vi "Parse JSON for Channels.vi"(7 "Settings(JSON)":string, 8 "error in":errorcluster) -> (0 "error out":errorcluster, 1 "Channel Paths":string[](array[string]), 2 "Channel TypeNames":string[](array[string]), 3 "Channel JSONs":string[](array[string]), 5 "Settings(JSON)":string)   [LabVIEW 2026, in "NIDMM Deployment Hooks.lvlib"]
uses:
  NIDMM Deployment Hooks.lvlib
  <vilib>/JDP Science/JSONtext/JSONtext.lvlib
  <vilib>/regexp/Match Regular Expression.xnode
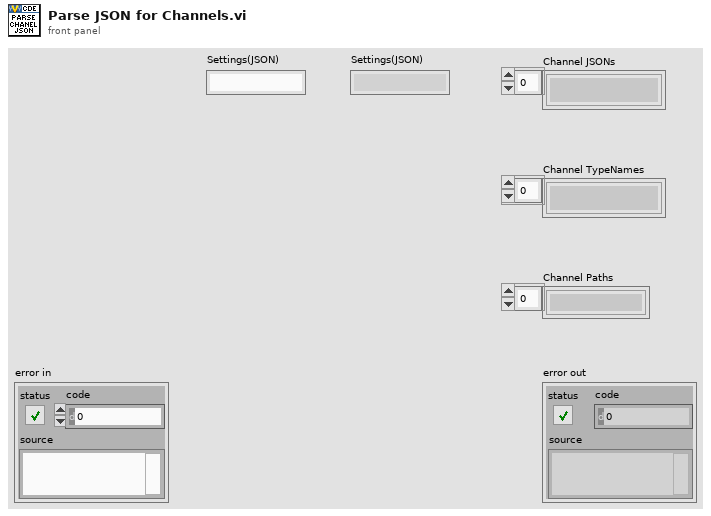
[diagram p1: front panel]
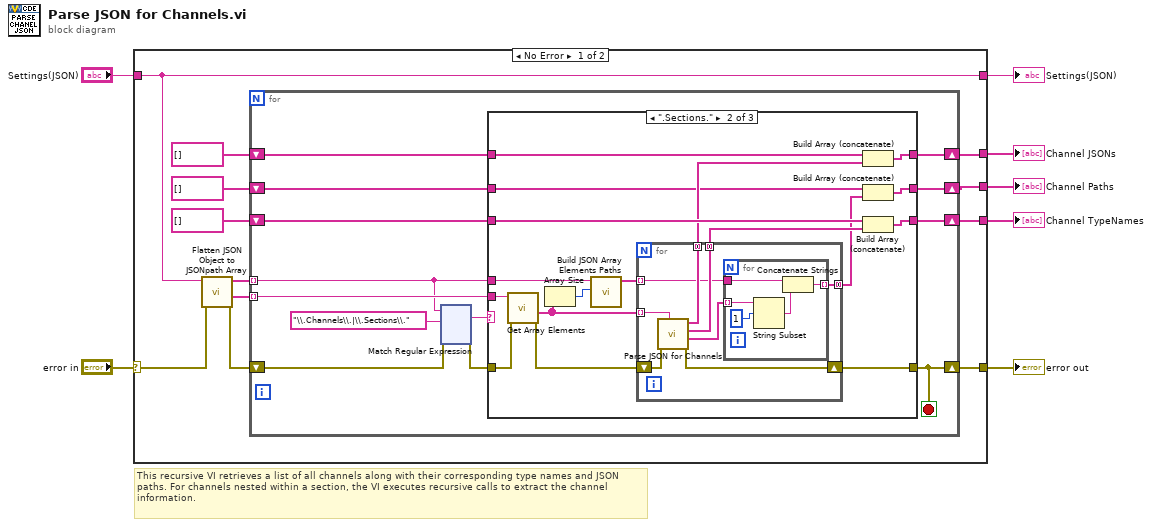
[diagram p0: block diagram]
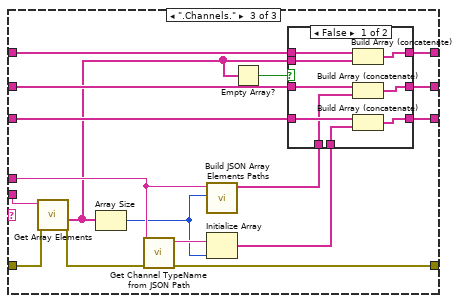
[diagram p3: hidden frame]
diagram:
  # "This recursive VI retrieves a list of all channels along with their corresponding type names and JSON paths. For channels nested within a section, the VI executes recursive calls to extract the channel information."
  n1 = case shown="No Error" "error in" {
    selector: "error in" -> [w18 w214]
    tunnel: [w17 w214] -> w7
    tunnel: "Settings(JSON)" -> [w10 w213]
    tunnel: [w12 _] -> w5
    tunnel: [w11 _] -> w4
    tunnel: [w10 w213] -> w2
    tunnel: [w8 _] -> w1
    frame No Error {
      n2 = call <vilib>:"Flatten JSON Object to JSONpath Array.vi"("error in (no error)"=w18, "JSON"=w10) -> ("error out"=w19:errorcluster, "<JSON>"=w15:string[], "$Paths"=w16:string[])  [unwired: 7 in]
      n3 = for {
        tunnel: w16 -> [w24] mode=indexing
        shift-right: [w28] -> w11
        shift-left: string[] [] ("<JSON>") -> [w29]
        tunnel: w15 -> [w27] mode=indexing
        shift-right: [w32] -> w17
        shift-left: w19 -> [w31]
        shift-right: [w25] -> w12
        shift-left: string[] [] -> [w26]
        shift-right: [w21] -> w8
        shift-left: string[] [] -> [w20]
        stop <- w32 stop-if-true
        n4 = xnode "Match Regular Expression"("input string"=w24, "regular expression"="\\.Channels\\.|\\.Sections\\.", "error in"=w31) -> ("whole match"=w22:string, "error out"=w30:errorcluster)  [unwired: 3 in, 3 out]
        n5 = case shown="\".Sections.\"" w22 {
          tunnel: [w36 w51 w81] -> w32
          tunnel: w29 -> [w34 w50 w69]
          tunnel: [w34 w45 w68] -> w28
          tunnel: w27 -> [_ w49 w78]
          tunnel: w26 -> [w35 w48 w79]
          tunnel: [w35 w47 w80] -> w25
          tunnel: w30 -> [w36 w53 w83]
          tunnel: w24 -> [_ w40 w72]
          tunnel: [w33 w42 w74] -> w21
          tunnel: w20 -> [w33 w43 w73]
          frame Default {
          }
          frame ".Sections." {
            n6 = call <vilib>:"Get Array Elements.vi"("error in (no error)"=w53, "JSON"=w49) -> ("error out"=w52:errorcluster, "<JSON>"=w41:string[])  [unwired: 7 in, 1 out]
            n7 = Array Size(array=w41) -> (size(s)=w39:i32)
            n8 = call "Build JSON Array Elements Paths.vi"("No Of Elements"=w39, "JSON Array Path"=w40) -> ("Paths"=w38:string[])  [unwired: 9 in]
            n9 = for {
              tunnel: w41 -> [w59] mode=indexing
              tunnel: [w57] -> w46 mode=concatenating
              tunnel: [w58] -> w44 mode=concatenating
              shift-right: [w60] -> w51
              shift-left: w52 -> [w61]
              tunnel: w38 -> [w55] mode=indexing
              tunnel: [w54] -> w37 mode=concatenating
              n10 = call "Parse JSON for Channels.vi"("Settings(JSON)"=w59, "error in"=w61) -> ("error out"=w60:errorcluster, "Channel Paths"=w56:string[], "Channel TypeNames"=w57:string[], "Channel JSONs"=w58:string[])  [unwired: 5 in, 1 out]
              n11 = for {
                tunnel: w56 -> [w66] mode=indexing
                tunnel: w55 -> [w64]
                tunnel: [w63] -> w54 mode=indexing
                n12 = String Subset(string=w66, offset (0)=1) -> (substring=w65:string)  [unwired: 1 in]
                n13 = Concatenate Strings(w64, w65) -> (w63:string)
              }
            }
            n14 = Build Array (concatenate)(w50, w44) -> (w45:string[])
            n15 = Build Array (concatenate)(w43, w37) -> (w42:string[])
            n16 = Build Array (concatenate)(w48, w46) -> (w47:string[])
          }
          frame ".Channels." {
            n17 = call <vilib>:"Get Array Elements.vi"("error in (no error)"=w83, "JSON"=w78) -> ("error out"=w82:errorcluster, "<JSON>"=w67:string[])  [unwired: 7 in, 1 out]
            n18 = Array Size(array=w67) -> (size(s)=w71:i32)
            n19 = call "Get Channel TypeName from JSON Path.vi"("error in"=w82, "Path"=w72) -> ("error out"=w81:errorcluster, "Type Name"=w75:string)  [unwired: 8 in]
            n20 = call "Build JSON Array Elements Paths.vi"("No Of Elements"=w71, "JSON Array Path"=w72) -> ("Paths"=w70:string[])  [unwired: 9 in]
            n21 = Initialize Array(w75, w71) -> (w76:string[])
            n22 = Empty Array?(array=w67) -> (empty?=w77:bool)
            n23 = case shown="False" w77 {
              tunnel: w76 -> [w87 _]
              tunnel: [w92 w95] -> w80
              tunnel: w79 -> [w91 w95]
              tunnel: [w90 w94] -> w74
              tunnel: w73 -> [w89 w94]
              tunnel: w70 -> [w88 _]
              tunnel: w69 -> [w86 w93]
              tunnel: [w85 w93] -> w68
              tunnel: w67 -> [w84 _]
              frame False {
                n24 = Build Array (concatenate)(w86, w84) -> (w85:string[])
                n25 = Build Array (concatenate)(w89, w88) -> (w90:string[])
                n26 = Build Array (concatenate)(w91, w87) -> (w92:string[])
              }
              frame True {
              }
            }
          }
        }
      }
    }
    frame Error {
    }
  }
  "error out" <- w7
  "Channel TypeNames" <- w5
  "Channel JSONs" <- w4
  "Settings(JSON)" <- w2
  "Channel Paths" <- w1
